vi "UV-VIS StartAcquisition.vi"(3 "error in (no error)":errorcluster, 5 "Detector in":refnum<class "CCD_camera.lvclass">) -> (0 "error out":errorcluster, 1 "DLL error code":u32, 2 "Detector out":refnum<class "CCD_camera.lvclass">)   [LabVIEW 2020, in "CCD_camera.lvclass"]
doc: "This function starts an acquisition. The status of the acquisition can be monitored via <B>GetStatus</B>.\n\n<B>Error codes:</B>\nDRV_SUCCESS - Acquisition started.\nDRV_NOT_INITIALIZED - System not initialized.\nDRV_ACQUIRING - Acquisition in progress.\nDRV_VXDNOTINSTALLED - VxD not loaded.\nDRV_ERROR_ACK - Unable to communicate with card.\nDRV_INIERROR - Error reading \"DETECTOR.INI\".\nDRV_ACQUISITION_ERRORS - Acquisition settings invalid.\nDRV_ERROR_PAGELOCK - Unable to allocate memory.\nDRV_INVALID_FILTER - Filter not available for current acquisition."
uses:
  CCD_camera.lvclass
  C:/dev/TRANCON/Classes/Detector/Detector.lvclass
  Detector.lvclass/Detector.ctl
  Detector.lvclass
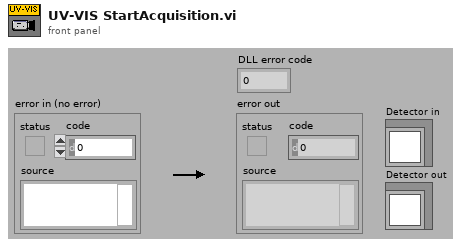
[diagram p1: front panel]
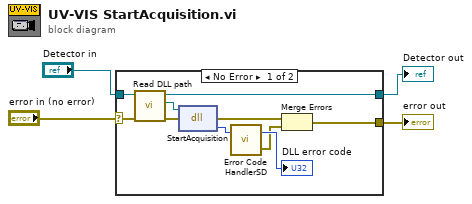
[diagram p0: block diagram]
diagram:
  n1 = case shown="No Error" "error in (no error)" {
    selector: "error in (no error)" -> [w9 w16]
    tunnel: [w11 w16] -> w3
    tunnel: [w5 w15] -> w2
    tunnel: "Detector in" -> [w7 w15]
    frame No Error {
      n2 = call "Read DLL path.vi"("error in (no error)"=w9, "Detector in"=w7) -> ("error out"=w8:errorcluster, "DLL path"=w10:path, "Detector out"=w5:refnum<class "CCD_camera.lvclass">)  [unwired: 7 in]
      n3 = dll-call lib="S:/TRANCON/DLL/Atmcd32d.dll" fn="StartAcquisition"(path in=w10, error in=w8) -> (error out=w6:errorcluster, "return type"=w14:u32)  [unwired: 1 in, 1 out]
      n4 = call "Error Code HandlerSD.vi"("DLL error code"=w14) -> ("error out"=w12:errorcluster, "dup DLL error code"=→"DLL error code":u32)  [unwired: 1 in]
      n5 = Merge Errors(w6, w12) -> (w11:errorcluster)
    }
    frame Error {
    }
  }
  "error out" <- w3
  "Detector out" <- w2
